vi "_Queue Create.vi"(9 "Queue jettl":refnum<class "Queue jettl.lvclass">, 10 "Alias":string) -> (3 "Queue Create Msg Strategy out":refnum<class "Queue Create Msg Strategy.lvclass">)   [LabVIEW 2021, in "jettl Msg Queue Create.lvlib"]
uses:
  jettl Msg Queue Create.lvlib
  Queue Create Msg Strategy/Queue Create Msg Strategy.lvclass
  jettl/Queue jettl/Queue jettl.lvclass
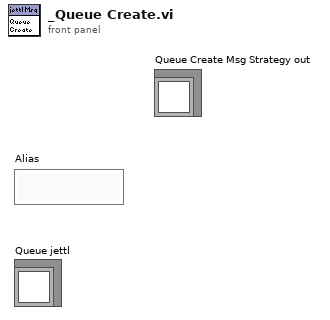
[diagram p1: front panel]
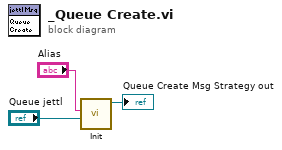
[diagram p0: block diagram]
diagram:
  n1 = call "Init.vi"("Queue jettl"="Queue jettl", "Alias"="Alias") -> ("Queue Create Msg Strategy out"=→"Queue Create Msg Strategy out":refnum<class "Queue Create Msg Strategy.lvclass">)  [unwired: 9 in]
